vi "Read PCBAID.vi"(11 "Error In":errorcluster) -> (4 "PCBAID":u8, 15 "Error Out":errorcluster)   [LabVIEW 2021, in "PCAN Reader.lvlib"]
doc: "Reads the IPC PCBAID based on the following hardcoded dbc definition:\n\nBO_ 2421161985 IPC_BootData_0: 8 IPC\n SG_ IPC_Boot_MetaVersion : 0|16@1+ (1,0) [0|65535] \"\" HC\n SG_ IPC_Boot_MCU_ID : 16|16@1+ (1,0) [0|65535] \"\" HC\n SG_ IPC_Boot_PCBA_ID : 32|16@1+ (1,0) [0|65535] \"\" HC\n SG_ IPC_Boot_Config_ID : 48|16@1+ (1,0) [0|65535] \"\" HC"
uses:
  PCAN Reader.lvlib
  <instrlib>/KDI Digital Instrumentation/API_for_PCAN_BASIC_FD/TPCANBaudrate.ctl
  <instrlib>/KDI Digital Instrumentation/API_for_PCAN_BASIC_FD/TPCANHandle.ctl
panel:
  in  "stop":bool
  # "Inputs"
  # "Outputs"
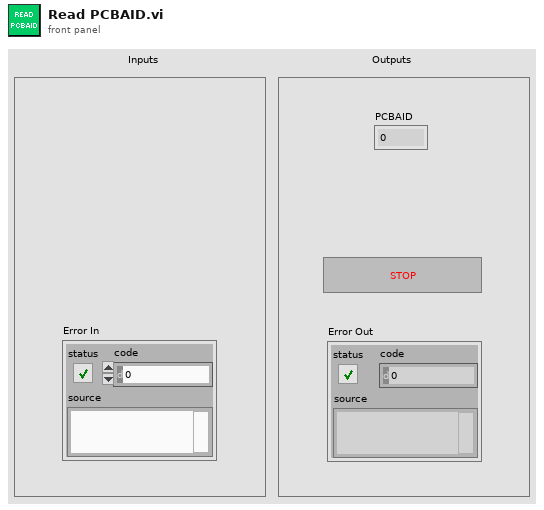
[diagram p1: front panel]
types:
  T1 = typedef "TPCANBaudrate.ctl" = enum16{"PCAN_BAUD_1M 0x0014", "PCAN_BAUD_800K 0x0016", "PCAN_BAUD_500K 0x001C", "PCAN_BAUD_250K 0x011C", "PCAN_BAUD_125K 0x031C", "PCAN_BAUD_100K 0x432F", "PCAN_BAUD_95K 0xC34E", "PCAN_BAUD_83K 0x852B", "PCAN_BAUD_50K 0x472F", "PCAN_BAUD_47K 0x1414", "PCAN_BAUD_33K 0x8B2F", "PCAN_BAUD_20K 0x532F", "PCAN_BAUD_10K 0x672F", "PCAN_BAUD_5K 0x7F7F", "User Baudrate"}
  T2 = typedef "TPCANHandle.ctl" = enum16{"PCAN_NONEBUS  0x000", "PCAN_ISABUS1  0x21", "PCAN_ISABUS2  0x22", "PCAN_ISABUS3  0x23", "PCAN_ISABUS4  0x24", "PCAN_ISABUS5  0x25", "PCAN_ISABUS6  0x26", "PCAN_ISABUS7  0x27", "PCAN_ISABUS8  0x28", "PCAN_DNGBUS1  0x31", "PCAN_PCIBUS1  0x41", "PCAN_PCIBUS1  0x42", "PCAN_PCIBUS1  0x43", "PCAN_PCIBUS1  0x44", "PCAN_PCIBUS1  0x45", "PCAN_PCIBUS1  0x46", "PCAN_PCIBUS1  0x47", "PCAN_PCIBUS1  0x48", "PCAN_PCIBUS1  0x409", "PCAN_PCIBUS1  0x40A", "PCAN_PCIBUS1  0x40B", "PCAN_PCIBUS1  0x40C", "PCAN_PCIBUS1  0x40D", "PCAN_PCIBUS1  0x40E", "PCAN_PCIBUS1  0x40F", "PCAN_PCIBUS1  0x410", "PCAN_USBBUS1  0x51", "PCAN_USBBUS2  0x52", "PCAN_USBBUS3  0x53", "PCAN_USBBUS4  0x54", "PCAN_USBBUS5  0x55", "PCAN_USBBUS6  0x56", "PCAN_USBBUS7  0x57", "PCAN_USBBUS8  0x58", "PCAN_USBBUS9  0x509", "PCAN_USBBUS10  0x50A", "PCAN_USBBUS11  0x50B", "PCAN_USBBUS12  0x50C", "PCAN_USBBUS13  0x50D", "PCAN_USBBUS14  0x50E", "PCAN_USBBUS15  0x50F", "PCAN_USBBUS16  0x510", "PCAN_PCCBUS1  0x61", "PCAN_PCCBUS2  0x62", "PCAN_LANBUS1  0x801", "PCAN_LANBUS2  0x802", "PCAN_LANBUS3  0x803", "PCAN_LANBUS4  0x804", "PCAN_LANBUS5  0x805", "PCAN_LANBUS6  0x806", "PCAN_LANBUS7  0x807", "PCAN_LANBUS8  0x808", "PCAN_LANBUS9  0x809", "PCAN_LANBUS10  0x80A", "PCAN_LANBUS11  0x80B", "PCAN_LANBUS12  0x80C", "PCAN_LANBUS13  0x80D", "PCAN_LANBUS14  0x80E", "PCAN_LANBUS15  0x80F", "PCAN_LANBUS16  0x810"}
  T3 = typedef "PCAN Reader.lvlib/PCANMessage.ctl" = cluster{"CAN_Message":T4, "TPCANTimestamp":T5}
  T4 = typedef "CAN MSG Cluster.ctl" = cluster{"ID":u32, "MSG type":u8, "DLC":u8, "DATA":u8[]}
  T5 = typedef "TPCANTimestamp.ctl" = cluster{"millis overflow":u16, "millis ":u32, "micros":u16}
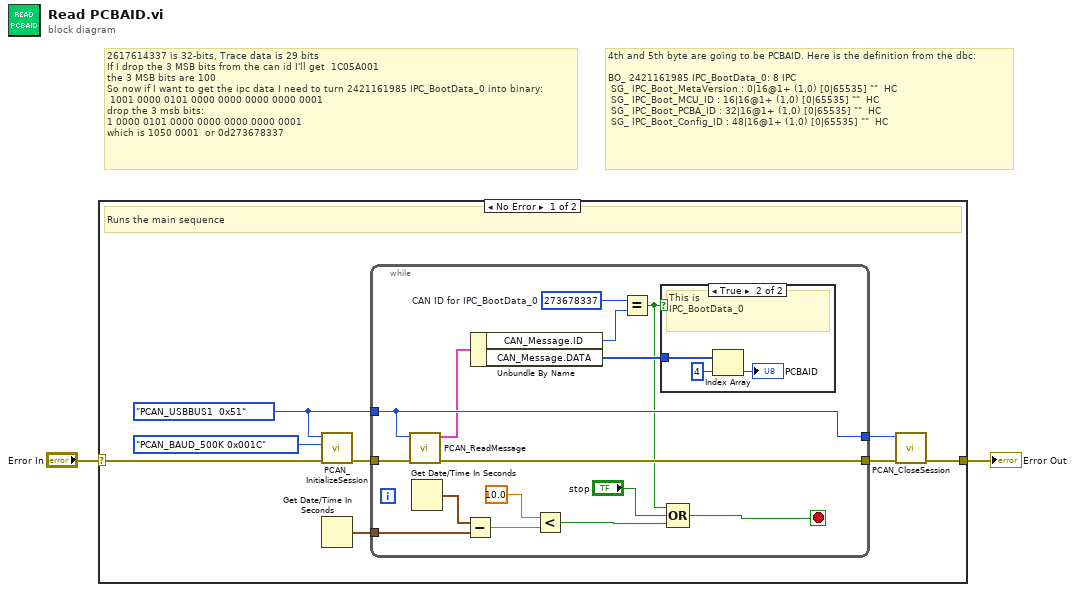
[diagram p0: block diagram]
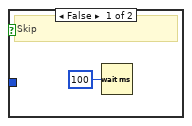
[diagram p2: hidden frame]
diagram:
  # "4th and 5th byte are going to be PCBAID. Here is the definition from the dbc:\n\nBO_ 2421161985 IPC_BootData_0: 8 IPC\n SG_ IPC_Boot_MetaVersion : 0|16@1+ (1,0) [0|65535] \"\"  HC\n SG_ IPC_Boot_MCU_ID : 16|16@1+ (1,0) [0|65535] \"\"  HC\n SG_ IPC_Boot_PCBA_ID : 32|16@1+ (1,0) [0|65535] \"\"  HC\n SG_ IPC_Boot_Config_ID : 48|16@1+ (1,0) [0|65535] \"\"  HC"
  # "2617614337 is 32-bits, Trace data is 29 bits\nIf I drop the 3 MSB bits from the can id I'll get  1C05A001\nthe 3 MSB bits are 100\nSo now if I want to get the ipc data I need to turn 2421161985 IPC_BootData_0 into binary:\n 1001 0000 0101 0000 0000 0000 0000 0001\ndrop the 3 msb bits:\n1 0000 0101 0000 0000 0000 0000 0001\nwhich is 1050 0001  or 0d273678337"
  n1 = case shown="No Error" "Error In" {
    selector: "Error In" -> [w10 w30]
    tunnel: [w9 w30] -> w1
    frame No Error {
      w5 = TPCANHandle."PCAN_USBBUS1  0x51" ("TPCANHandle")
      # "Runs the main sequence"
      n2 = call "PCAN_InitializeSession.vi"("error in (no error)"=w10, "TPCANBaudrate"=TPCANBaudrate."PCAN_BAUD_500K 0x001C", "TPCANHandle"=w5) -> ("error out"=w7:errorcluster)  [unwired: 8 in]
      n3 = Get Date/Time In Seconds() -> (seconds since 1Jan1904=w3:timestamp)
      n4 = while {
        tunnel: w7 -> [w25]
        tunnel: [w24] -> w6
        tunnel: w5 -> [w23]
        tunnel: [w23] -> w4
        tunnel: w3 -> [w17]
        stop <- w12 stop-if-true
        w19 = u32 273678337  # CAN ID for IPC_BootData_0
        n5 = call "PCAN_ReadMessage.vi"("error in (no error)"=w25, "TPCANHandle"=w23) -> ("error out"=w24:errorcluster, "Message"=w21:T3)  [unwired: 7 in, 1 out]
        n6 = Get Date/Time In Seconds() -> (seconds since 1Jan1904=w18:timestamp)
        n7 = Subtract(x=w18, y=w17) -> (x-y=w16:dbl)
        n8 = Unbundle By Name(w21) -> ("CAN_Message.ID"=w20:u32, "CAN_Message.DATA"=w22:u8[])
        n9 = Less?(x=10.0, y=w16) -> (x < y?=w14:bool)
        n10 = Equal?(x=w19, y=w20) -> (x = y?=w11:bool)
        n11 = case shown="True" w11 {
          tunnel: w22 -> [_ w29]
          frame False {
            # "Skip"
            n12 = Wait (ms)(milliseconds to wait=u32 100) -> ()  [unwired: 1 out]
          }
          frame True {
            # "This is\nIPC_BootData_0"
            n13 = Index Array(array=w29, index=4) -> (element=→"PCBAID":u8)
          }
        }
        n14 = Compound Arithmetic op=OR(w11, "stop", w14) -> (w12:bool)
      }
      n15 = call "PCAN_CloseSession.vi"("error in (no error)"=w6, "TPCANHandle"=w4) -> ("error out"=w9:errorcluster)  [unwired: 9 in]
    }
    frame Error {
      # "Can't start due to error"
    }
  }
  "Error Out" <- w1
